vi "Insert Subpanel.vi"(8 "Error In":errorcluster, 11 "VI Refnum":refnum<vi>) -> (0 "Error Out":errorcluster)   [LabVIEW 2019, in "Controller.lvlib"]
uses:
  Controller.lvlib
  Queues/Queues.lvlib
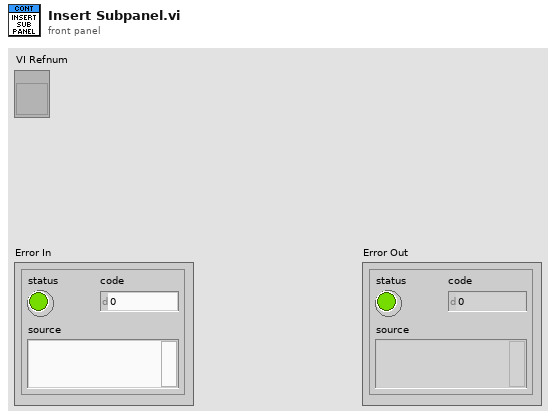
[diagram p1: front panel]
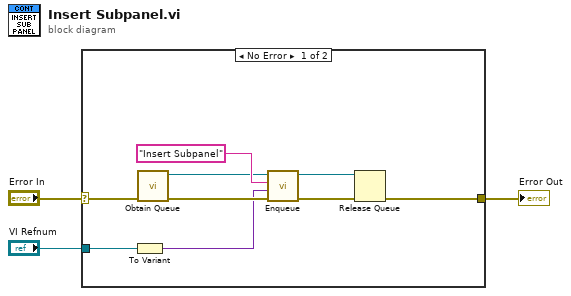
[diagram p0: block diagram]
diagram:
  n1 = case shown="No Error" "Error In" {
    selector: "Error In" -> [w11 w13]
    tunnel: [w6 w13] -> w3
    tunnel: "VI Refnum" -> [w5 _]
    frame No Error {
      n2 = To Variant(anything=w5) -> (Variant=w4:variant)
      n3 = call "Obtain Queue.vi"("Error In"=w11) -> ("Error Out"=w10:errorcluster, "Queue out"=w9:refnum<queue>)  [unwired: 9 in]
      n4 = call "Enqueue.vi"("Error In"=w10, "Data"=w4, "State"="Insert Subpanel", "Queue in"=w9) -> ("Error Out"=w8:errorcluster, "Queue out"=w7:refnum<queue>)  [unwired: 6 in]
      n5 = Release Queue(queue=w7, error in (no error)=w8) -> (error out=w6:errorcluster)  [unwired: 1 in, 2 out]
    }
    frame Error {
    }
  }
  "Error Out" <- w3
